vi "adam-sample-thermocouples.vi"(7 "Thermocouples":T1, 8 "error in (no error)":errorcluster, 11 "VISA Refnum in":refnum<visa-resource-name>) -> (0 "error out":errorcluster, 1 "status":string, 2 "read buffer":string, 3 "VISA Refnum out":refnum<visa-resource-name>, 4 "acknowledge char":string, 5 "Thermocouples out":T1)   [LabVIEW 2024]
uses:
  controls/depreciated/thermocouple-data-cluster.ctl
panel:
  in  "chassis slot":u8
  in  "ADAM-5000: Chassis ID":u8=1
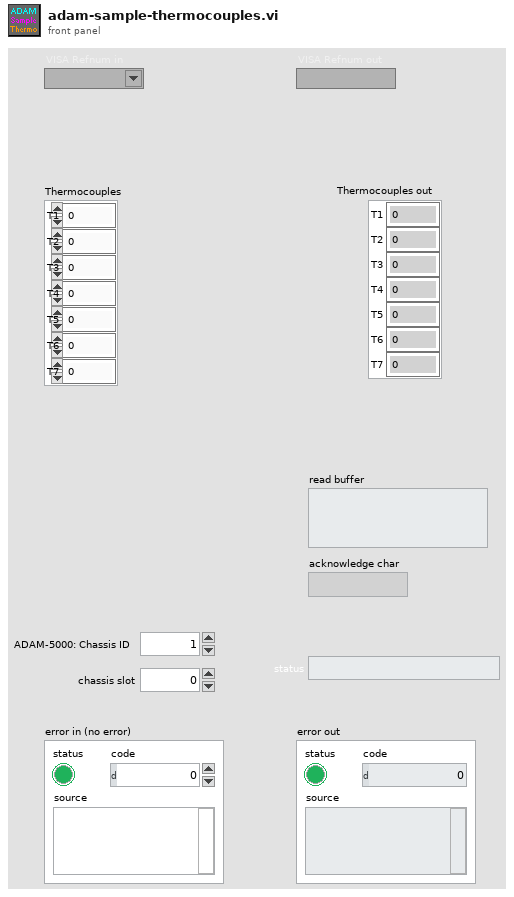
[diagram p1: front panel]
types:
  T1 = typedef "thermocouple-data-cluster.ctl" = cluster{"T1":dbl, "T2":dbl, "T3":dbl, "T4":dbl, "T5":dbl, "T6":dbl, "T7":dbl}
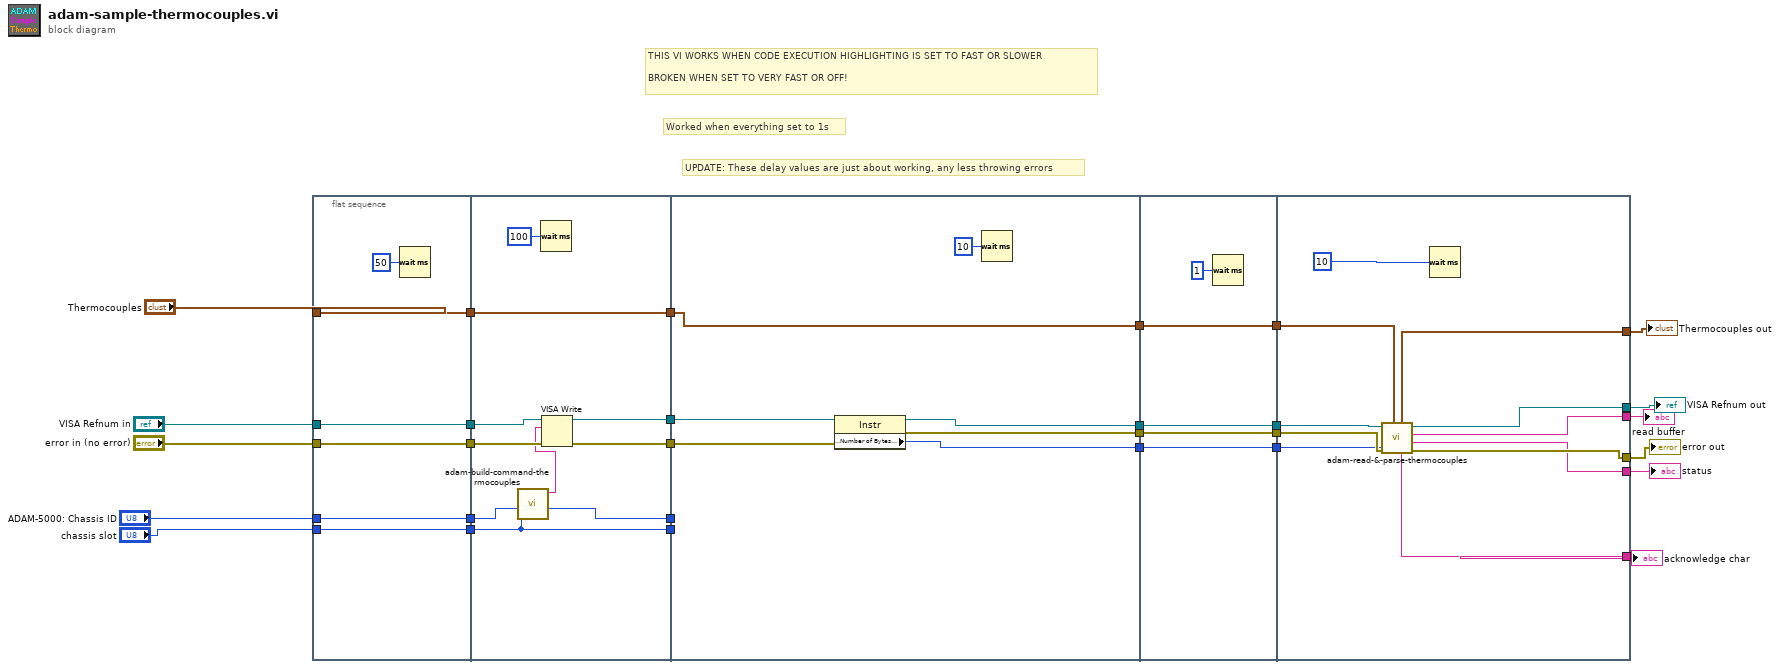
[diagram p0: block diagram]
diagram:
  # "UPDATE: These delay values are just about working, any less throwing errors"
  # "Worked when everything set to 1s"
  # "THIS VI WORKS WHEN CODE EXECUTION HIGHLIGHTING IS SET TO FAST OR SLOWER\n\nBROKEN WHEN SET TO VERY FAST OR OFF!"
  n1 = flat-sequence {
    tunnel: "Thermocouples" -> [w31]
    tunnel: "ADAM-5000: Chassis ID" -> [w32]
    tunnel: "chassis slot" -> [w33]
    tunnel: "VISA Refnum in" -> [w34]
    tunnel: "error in (no error)" -> [w35]
    tunnel: [w35] -> w7
    tunnel: [w34] -> w6
    tunnel: [w33] -> w5
    tunnel: [w32] -> w4
    tunnel: [w31] -> w3
    tunnel: [w43] -> w10
    tunnel: [w42] -> w9
    tunnel: [w41] -> w8
    tunnel: w7 -> [w44]
    tunnel: w6 -> [w38]
    tunnel: w5 -> [w43]
    tunnel: w4 -> [w42]
    tunnel: w3 -> [w41]
    tunnel: [w39] -> w2
    tunnel: [w37] -> w1
    tunnel: [w51] -> w29
    tunnel: [w50] -> w28
    tunnel: [w49] -> w27
    tunnel: [w48] -> w11
    tunnel: w10 -> [_]
    tunnel: w9 -> [_]
    tunnel: w8 -> [w48]
    tunnel: w2 -> [w46]
    tunnel: w1 -> [w45]
    tunnel: w29 -> [w56]
    tunnel: w28 -> [w55]
    tunnel: w27 -> [w54]
    tunnel: [w56] -> w26
    tunnel: [w55] -> w25
    tunnel: [w54] -> w24
    tunnel: [w52] -> w12
    tunnel: w11 -> [w52]
    tunnel: w26 -> [w67]
    tunnel: w25 -> [w65]
    tunnel: w24 -> [w66]
    tunnel: [w64] -> w18
    tunnel: [w63] -> w17
    tunnel: [w62] -> w14
    tunnel: [w61] -> w16
    tunnel: [w60] -> w15
    tunnel: [w59] -> w13
    tunnel: w12 -> [w58]
    frame #0 {
      n2 = Wait (ms)(milliseconds to wait=u32 50) -> ()  [unwired: 1 out]
    }
    frame #1 {
      n3 = call "adam-build-command-thermocouples.vi"("chassis slot"=w43, "ADAM-5000: Chassis ID"=w42) -> ("Command Out"=w40:string)  [unwired: 9 in]
      n4 = Wait (ms)(milliseconds to wait=u32 100) -> ()  [unwired: 1 out]
      n5 = VISA Write(VISA resource name=w38, write buffer=w40, error in (no error)=w44) -> (VISA resource name out=w37:refnum<visa-resource-name>, error out=w39:errorcluster)  [unwired: 1 out]
    }
    frame #2 {
      n6 = property class="Instr"(reference=w45, error in=w46) -> (reference out=w50:refnum<visa-resource-name>, error out=w51:errorcluster, "Serial Settings:Number of Bytes at Serial Port"=w49:u32)
      n7 = Wait (ms)(milliseconds to wait=u32 10) -> ()  [unwired: 1 out]
    }
    frame #3 {
      n8 = Wait (ms)(milliseconds to wait=u32 1) -> ()  [unwired: 1 out]
    }
    frame #4 {
      n9 = call "adam-read-&-parse-thermocouples.vi"("Thermocouples in"=w58, "error in (no error)"=w67, "Bytes at Port"=w66, "VISA Refnum in"=w65) -> ("error out"=w64:errorcluster, "status  out"=w63:string, "read buffer"=w62:string, "VISA Refnum out"=w61:refnum<visa-resource-name>, "acknowledge char"=w60:string, "Thermocouples out"=w59:T1)  [unwired: 2 in]
      n10 = Wait (ms)(milliseconds to wait=u32 10) -> ()  [unwired: 1 out]
    }
  }
  "status" <- w17
  "error out" <- w18
  "VISA Refnum out" <- w16
  "Thermocouples out" <- w13
  "read buffer" <- w14
  "acknowledge char" <- w15
